vi "FTW-Message-Request-WriteResponse.vi"(8 "error in":errorcluster, 9 "Response Body":string, 11 "FTW Incoming Request":refnum<class "FTW-Message-IncomingRequest.lvclass">) -> (0 "error out":errorcluster, 3 "FTW Incoming Request out":refnum<class "FTW-Message-IncomingRequest.lvclass">)   [LabVIEW 2013, in "FTW-Message-IncomingRequest.lvclass"]
uses:
  FTW-Message-IncomingRequest.lvclass
  FTW-Message-IncomingRequest.lvclass/FTW-Message-IncomingRequest.ctl
panel:
  # "Inputs"
  # "Outputs"
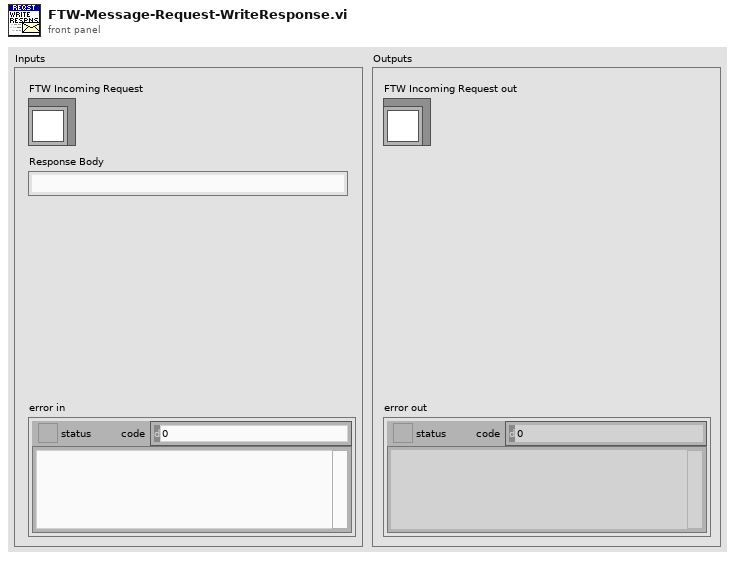
[diagram p1: front panel]
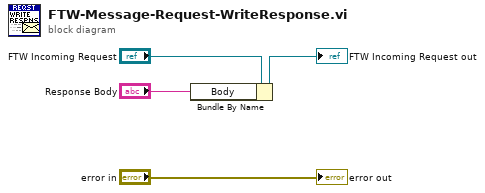
[diagram p0: block diagram]
diagram:
  n1 = Bundle By Name(cluster="FTW Incoming Request", "Body"="Response Body") -> (→"FTW Incoming Request out":refnum<class "FTW-Message-IncomingRequest.lvclass">)
  "error out" <- "error in"
